vi "ManipWaitForTeleOp.vi"() -> (0 "Error Out":errorcluster, 1 "Advance Trigger":bool)   [LabVIEW 2023]
doc: "This VI pauses the manipulator sequencer until the driver presses the \"advance system check\" button on the joystick, the joystick will rumble while waiting for the button."
uses:
  <vilib>/Rock Robotics/WPI/DriverStation/WPI_DriverStationRobotMode2.ctl
  GlobalDriverStationData.vi
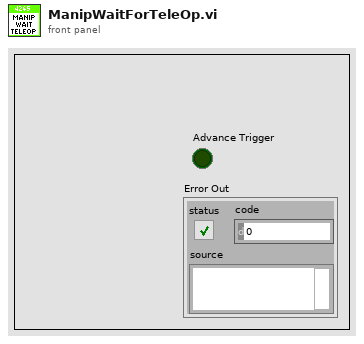
[diagram p1: front panel]
types:
  T1 = typedef "WPI_DriverStationRobotMode2.ctl" = enum16{"Autonomous Disabled", "Autonomous Enabled", "Teleop Disabled", "Teleop Enabled", "Disconnected", "Finish", "Test Disabled", "Test Enabled", "Emergency Stopped"}
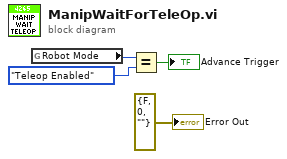
[diagram p0: block diagram]
diagram:
  n1 = global read "GlobalDriverStationData.vi" "Robot Mode"() -> (w2:T1)
  n2 = Equal?(x=w2, y=WPI_DriverStationRobotMode2."Teleop Enabled") -> (x = y?=→"Advance Trigger":bool)
  "Error Out" <- errorcluster {"status"=FALSE, "code"=0, "source"=""} ("error IO")
